vi "Agilent U2000 Series Range Test.vi"() -> ()   [LabVIEW 2018]
doc: "This example shows how to configure a range and check that the acquired measurements are within that range using the VIs of the driver.\n\nNote:\nThis example is not applicable for U2021/2XA."
uses:
  Agilent U2000 Series.lvlib
panel:
  out "Out of Range":bool
  in  "Lower Limit (-90.0 dBm)":dbl=-90.0 format="%#.6g"
  in  "Upper Limit (90.0 dBm)":dbl=90.0 format="%#.6g"
  in  "Timeout (10000 ms)":u32=10000
  out "Measurement":dbl
  in  "VISA resource name":refnum<visa-resource-name>
  # "(c) 2011-2015 National Instruments.  ALL RIGHTS RESERVED."
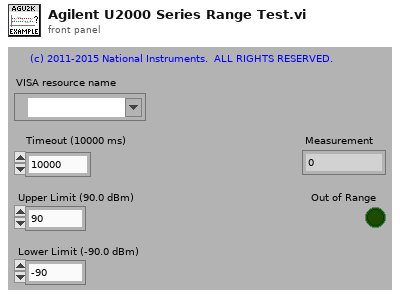
[diagram p1: front panel]
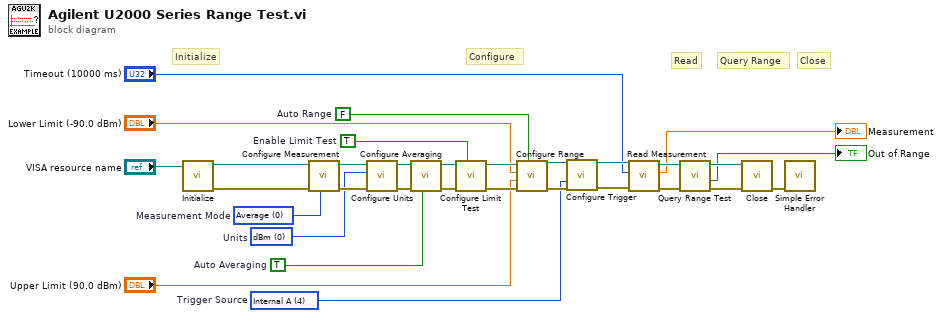
[diagram p0: block diagram]
diagram:
  w1 = 0 items=["dBm", "Watts"]  # Units
  w9 = TRUE  # Enable Limit Test
  w11 = 4 items=["Bus", "External", "Hold", "Immediate", "Internal A"]  # Trigger Source
  w4 = 0 items=["Average", "Normal"]  # Measurement Mode
  w3 = TRUE  # Auto Averaging
  w10 = FALSE  # Auto Range
  # "Query Range"
  # "Close"
  # "Read"
  # "Configure"
  # "Initialize"
  n1 = call "Initialize.vi"("VISA resource name"="VISA resource name") -> ("error out"=w5:errorcluster, "VISA resource name out"=w6:refnum<visa-resource-name>)  [unwired: 3 in, 6 out]
  n2 = call "Configure Measurement.vi"("Measurement Function (0: Average)"=w4, "error in (no error)"=w5, "VISA resource name"=w6) -> ("error out"=w30:errorcluster, "VISA resource name out"=w29:refnum<visa-resource-name>)  [unwired: 7 in]
  n3 = call "Configure Units.vi"("error in (no error)"=w30, "Units (0: dBm)"=w1, "VISA resource name"=w29) -> ("error out"=w28:errorcluster, "VISA resource name out"=w27:refnum<visa-resource-name>)  [unwired: 1 in, 6 out]
  n4 = call "Configure Averaging.vi"("Auto Averaging (T: Enable)"=w3, "error in (no error)"=w28, "VISA resource name"=w27) -> ("error out"=w26:errorcluster, "VISA resource name out"=w25:refnum<visa-resource-name>)  [unwired: 7 in]
  n5 = call "Configure Limit Test.vi"("Limit Test (T: Enable)"=w9, "error in (no error)"=w26, "VISA resource name"=w25) -> ("error out"=w24:errorcluster, "VISA resource name out"=w23:refnum<visa-resource-name>)  [unwired: 2 in, 5 out]
  n6 = call "Configure Range.vi"("Auto Range (T: Enable)"=w10, "error in (no error)"=w24, "Upper Limit (90 dBm)"="Upper Limit (90.0 dBm)", "Lower Limit (-90 dBm)"="Lower Limit (-90.0 dBm)", "VISA resource name"=w23) -> ("error out"=w12:errorcluster, "VISA resource name out"=w2:refnum<visa-resource-name>)  [unwired: 5 in]
  n7 = call "Configure Trigger.vi"("VISA resource name"=w2, "Trigger Source (3: Immediate)"=w11, "error in (no error)"=w12) -> ("VISA resource name out"=w21:refnum<visa-resource-name>, "error out"=w22:errorcluster)  [unwired: 5 in, 6 out]
  n8 = call "Read Measurement.vi"("error in (no error)"=w22, "Timeout (10000 ms)"="Timeout (10000 ms)", "VISA resource name"=w21) -> ("error out"=w20:errorcluster, "Measurement"=→"Measurement":dbl, "VISA resource name out"=w19:refnum<visa-resource-name>)  [unwired: 6 out]
  n9 = call "Query Range Test.vi"("error in (no error)"=w20, "VISA resource name"=w19) -> ("error out"=w16:errorcluster, "Limit Failure?"=→"Out of Range":bool, "VISA resource name out"=w17:refnum<visa-resource-name>)  [unwired: 1 in, 6 out]
  n10 = call "Close.vi"("error in (no error)"=w16, "VISA resource name"=w17) -> ("error out"=w18:errorcluster)  [unwired: 9 out]
  n11 = call <vilib>:"Simple Error Handler.vi"("error in (no error)"=w18) -> ()  [unwired: 1 in, 8 out]
